vi "Revision Query.vi"(8 "error in (no error)":errorcluster, 11 "Honeywell Compass HMC6343":refnum<class "Honeywell Compass HMC6343.lvclass">) -> (0 "error out":errorcluster, 1 "Device Serial Number":u16, 2 "Software Version Number":u8, 3 "Honeywell Compass HMC6343 out":refnum<class "Honeywell Compass HMC6343.lvclass">, 4 "Package Time":cluster{"Year":u8, "Week":u8})   [LabVIEW 2019, in "Honeywell Compass HMC6343.lvclass"]
doc: "Reads the information of this device, including Software Version Number, Device Serial Number and Package Time."
uses:
  Honeywell Compass HMC6343.lvclass
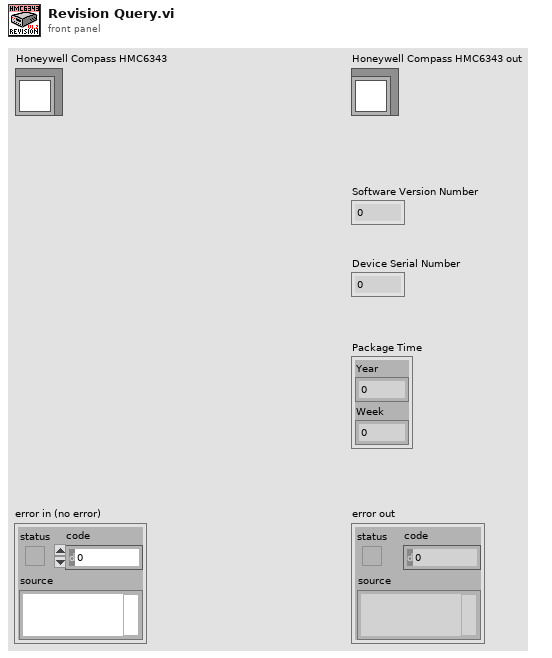
[diagram p1: front panel]
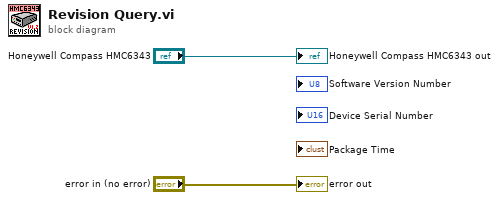
[diagram p0: block diagram]
diagram:
  "error out" <- "error in (no error)"
  "Honeywell Compass HMC6343 out" <- "Honeywell Compass HMC6343"
